vi "Check if Position Passed.vi"(6 "previous position (n-1)":u16, 7 "trigger position":u16, 9 "rotated forward":bool, 10 "cycle wrapped":bool, 11 "position":u16) -> (3 "trigger":bool)   [LabVIEW 2015, in "Engine Simulation Toolkit.lvlib"]
uses:
  Engine Simulation Toolkit.lvlib
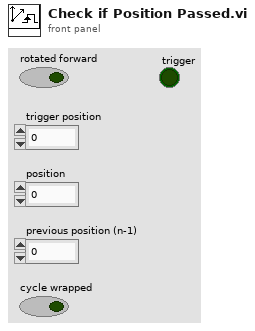
[diagram p1: front panel]
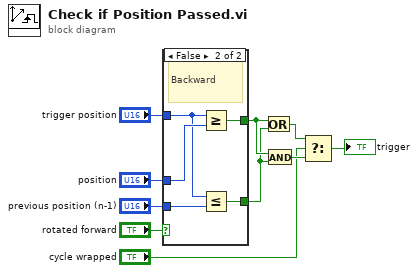
[diagram p0: block diagram]
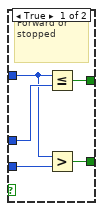
[diagram p2: hidden frame]
diagram:
  n1 = case shown="False" "rotated forward" {
    tunnel: "position" -> [w15 w20]
    tunnel: "previous position (n-1)" -> [w13 w18]
    tunnel: "trigger position" -> [w14 w19]
    tunnel: [w12 w17] -> w4
    tunnel: [w11 w16] -> w3
    frame True {
      # "Forward or stopped"
      n2 = Less Or Equal?(x=w14, y=w15) -> (x <= y?=w12:bool)
      n3 = Greater?(x=w14, y=w13) -> (0:w11:bool)
    }
    frame False {
      # "Backward"
      n4 = Greater Or Equal?(x=w19, y=w20) -> (x >= y?=w17:bool)
      n5 = Less Or Equal?(x=w19, y=w18) -> (x <= y?=w16:bool)
    }
  }
  n6 = Or(x=w4, y=w3) -> (x .or. y?=w7:bool)
  n7 = And(x=w4, y=w3) -> (x .and. y?=w6:bool)
  n8 = Select(t=w7, s="cycle wrapped", f=w6) -> (s? t:f=→"trigger":bool)
